vi "Day 20-Remove Padding.vi"(11 "Array in":bool[][](array[boolean])) -> (3 "Array out":bool[][](array[boolean]))   [LabVIEW 2021]
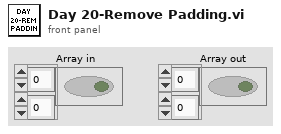
[diagram p1: front panel]
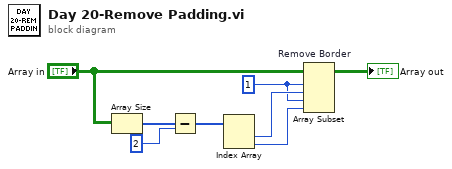
[diagram p0: block diagram]
diagram:
  w1 = 1
  n1 = Array Size(array="Array in") -> (size(s)=w3:i32[])
  n2 = Subtract(x=w3, y=2) -> (x-y=w6:i32[])
  n3 = Index Array(array=w6) -> (element #1=w7:i32, element #2=w8:i32)  [unwired: 2 in]
  n4 = Array Subset "Remove Border"(array="Array in", index (row)=w1, length (row)=w7, index (col)=w1, length (col)=w8) -> (→"Array out":bool[][])
